vi "Timer FGV.vi"(11 "Enum":T1) -> (3 "Elapsed Time":dbl)   [LabVIEW 2017, in "controllerLibrary.lvlib"]
uses:
  controllerLibrary.lvlib
  Controls/timer control.ctl
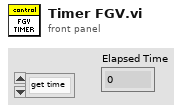
[diagram p1: front panel]
types:
  T1 = typedef "controllerLibrary.lvlib/timer control.ctl" = enum16{"get time", "set time"}
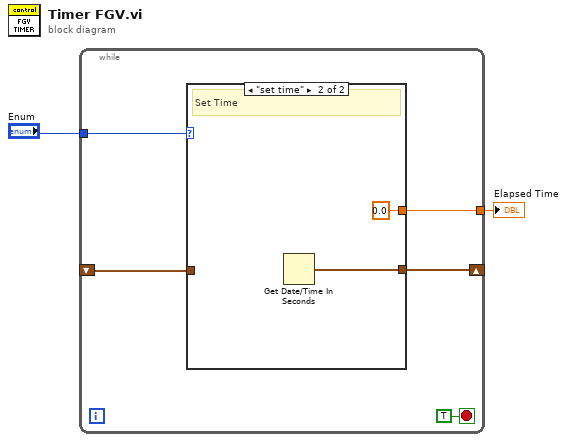
[diagram p0: block diagram]
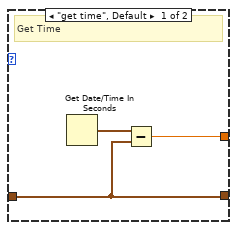
[diagram p2: hidden frame]
diagram:
  n1 = while {
    tunnel: "Enum" -> [w6]
    shift-right: [w5] -> _
    shift-left: _ -> [w4]
    tunnel: [w3] -> w2
    stop <- TRUE stop-if-true
    n2 = case shown="\"set time\"" w6 {
      tunnel: [w9 w12] -> w5
      tunnel: w4 -> [w9 _]
      tunnel: [w8 0.0] -> w3
      frame "get time", Default {
        # "Get Time"
        n3 = Get Date/Time In Seconds() -> (seconds since 1Jan1904=w10:timestamp)
        n4 = Subtract(x=w10, y=w9) -> (x-y=w8:dbl)
      }
      frame "set time" {
        # "Set Time"
        n5 = Get Date/Time In Seconds() -> (seconds since 1Jan1904=w12:timestamp)
      }
    }
  }
  "Elapsed Time" <- w2
